vi "HealthCheck.vi"() -> ()   [LabVIEW 2017]
panel:
  out "Right Velocity":sgl
  out "BR Count":u8
  out "FR Count":u8
  in  "FPGA_Ref":T1
  in  "LOG":bool
  out "Reserve Battery Voltage 2":string
  out "IMU Z Accel":string
  out "IMU Y Accel":string
  out "IMU X Accel":string
  out "Light Sensor Right":string
  out "Light Sensor Left":string
  out "IR 4":string
  out "IR 3":string
  out "PCS Temp 2":string
  out "Pn High Pressure":string
  out "Pn Low Pressure":string
  out "Ambient Pressure":string
  out "Highest Battery Temp":string
  out "Reserve Battery Voltage":string
  out "Primary Battery 2 Voltage":string
  out "Primary Battery 1 Voltage":string
  in  "IMU_Ref":T2
  out "Y/N? 2":bool
  out "Ambient P Max 2":dbl
  out "Ambient P 2":dbl
  out "Downstream Right":dbl
  out "Y/N?":bool
  out "IMU Z Max":dbl
  out "IMU Z":dbl
  out "IMU Z Min":dbl
  out "Y/N? 3":bool
  out "IMU Y Max":dbl
  out "IMU Y":dbl
  out "IMU Y Min":dbl
  out "Y/N? 4":bool
  out "IMU X Max":dbl
  out "IMU X":dbl
  out "IMU X Min":dbl
  out "HP":dbl
  out "Y/N? 5":bool
  out "LS FR Max":dbl
  out "LS Right":dbl
  out "LS FR Min":dbl
  out "Y/N? 6":bool
  out "LS FL Max":dbl
  out "LS Left":dbl
  out "LS FL Min":dbl
  out "Y/N? 7":bool
  out "IR 2 Max":dbl
  out "IR 2":dbl
  out "IR 2 Min":dbl
  out "Y/N? 8":bool
  out "IR 1 Max":dbl
  out "IR 1":dbl
  out "IR 1 Min":dbl
  out "Y/N? 9":bool
  out "Ambient P Max":dbl
  out "Ambient P":dbl
  out "Ambient P Min":dbl
  out "Y/N? 10":bool
  out "LP Max":dbl
  out "LP":dbl
  out "LP1 Min":dbl
  out "Y/N? 11":bool
  out "HP Max":dbl
  out "HP Min":dbl
  out "Y/N? 12":bool
  out "PCS Temp Max":dbl
  out "PCS Temp":dbl
  out "PCS Temp Min":dbl
  out "Y/N? 13":bool
  out "HBT Max":dbl
  out "HBT":dbl
  out "HBT Min":dbl
  out "Y/N? 14":bool
  out "RBV Max":dbl
  out "RBV":dbl
  out "RBV Min":dbl
  out "Y/N? 15":bool
  out "PB2V Max":dbl
  out "PB2 V":dbl
  out "PB2V Min":dbl
  out "Y/N? 16":bool
  out "PB1V Max":dbl
  out "PB1V":dbl
  out "PB1V Min":dbl
  # "Sensor"
  # "Min"
  # "Actual"
  # "Max"
  # "Status"
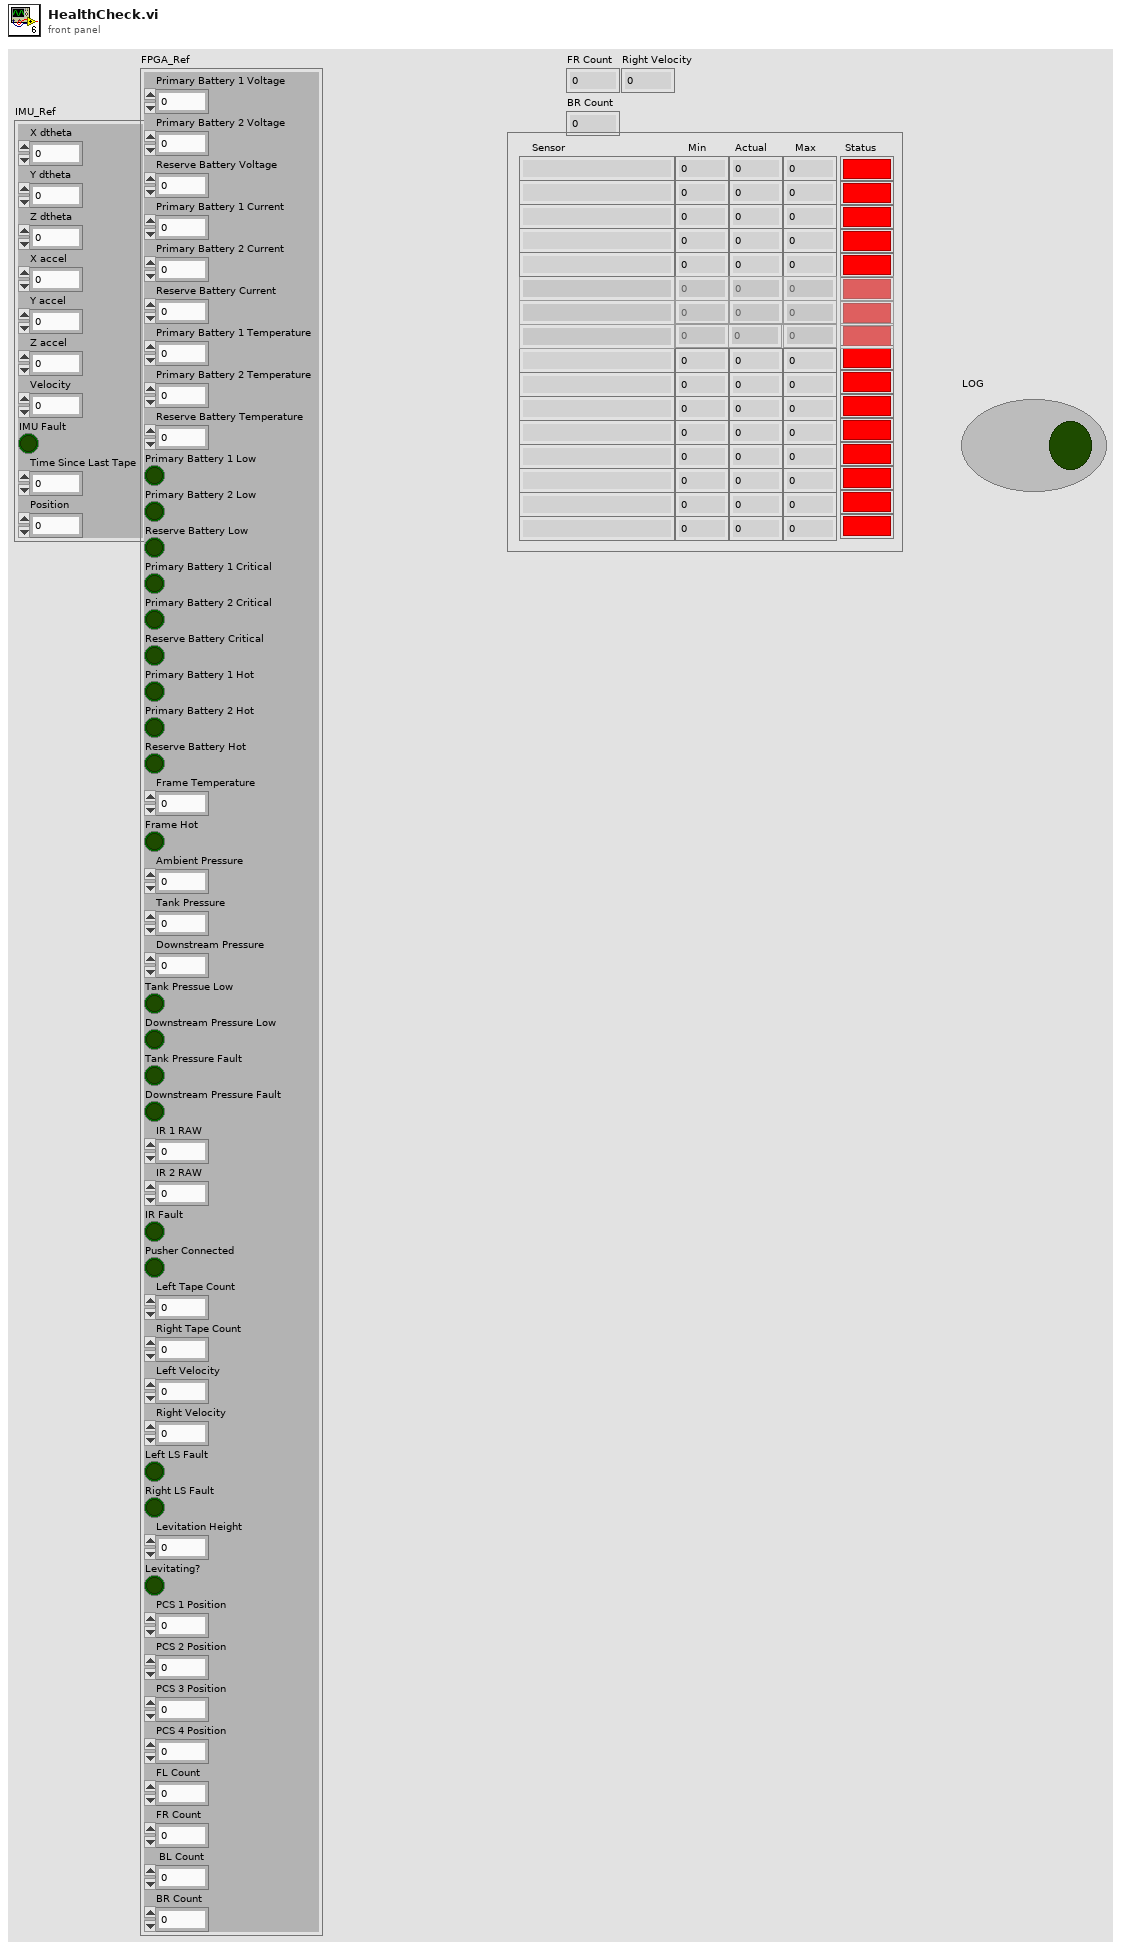
[diagram p1: front panel]
types:
  T1 = cluster{"Primary Battery 1 Voltage":sgl, "Primary Battery 2 Voltage":sgl, "Reserve Battery Voltage":sgl, "Primary Battery 1 Current":sgl, "Primary Battery 2 Current":sgl, "Reserve Battery Current":sgl, "Primary Battery 1 Temperature":sgl, "Primary Battery 2 Temperature":sgl, "Reserve Battery Temperature":sgl, "Primary Battery 1 Low":bool, "Primary Battery 2 Low":bool, "Reserve Battery Low":bool, "Primary Battery 1 Critical":bool, "Primary Battery 2 Critical":bool, "Reserve Battery Critical":bool, "Primary Battery 1 Hot":bool, "Primary Battery 2 Hot":bool, "Reserve Battery Hot":bool, "Frame Temperature":sgl, "Frame Hot":bool, "Ambient Pressure":sgl, "Tank Pressure":sgl, "Downstream Pressure":sgl, "Tank Pressue Low":bool, "Downstream Pressure Low":bool, "Tank Pressure Fault":bool, "Downstream Pressure Fault":bool, "IR 1 RAW":sgl, "IR 2 RAW":sgl, "IR Fault":bool, "Pusher Connected":bool, "Left Tape Count":u32, "Right Tape Count":u32, "Left Velocity":sgl, "Right Velocity":sgl, "Left LS Fault":bool, "Right LS Fault":bool, "Levitation Height":sgl, "Levitating?":bool, "PCS 1 Position":sgl, "PCS 2 Position":sgl, "PCS 3 Position":sgl, "PCS 4 Position":sgl, "FL Count":u8, "FR Count":u8, " BL Count":u8, "BR Count":u8}
  T2 = cluster{"X dtheta":sgl, "Y dtheta":sgl, "Z dtheta":sgl, "X accel":sgl, "Y accel":sgl, "Z accel":sgl, "Velocity":sgl, "IMU Fault":bool, "Time Since Last Tape":sgl, "Position":sgl}
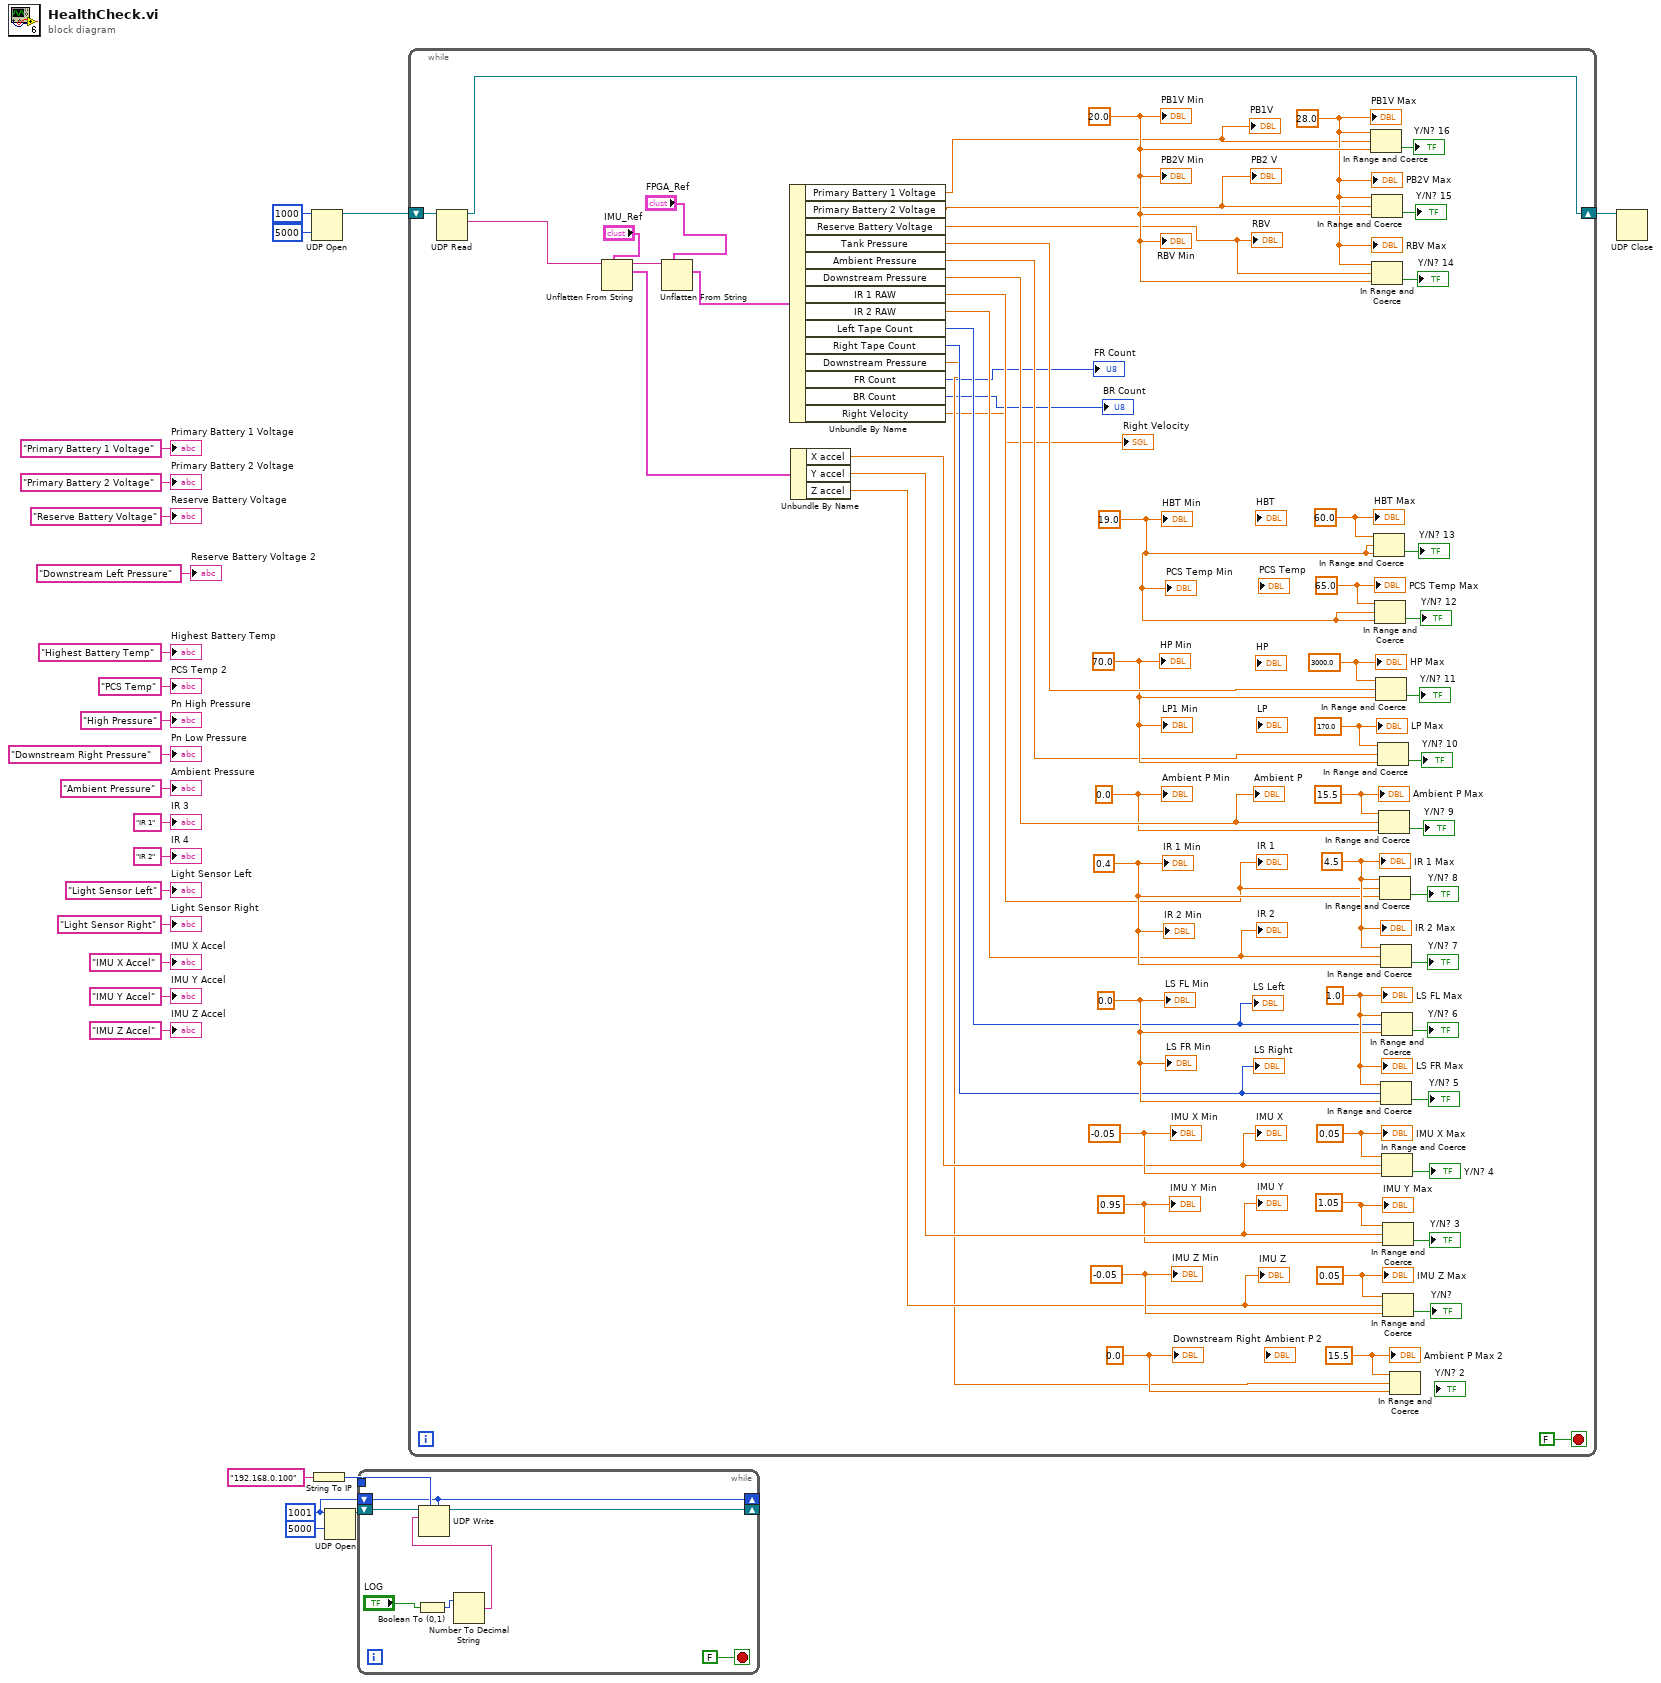
[diagram p0: block diagram]
diagram:
  w4 = u16 1001 ("port")
  n1 = UDP Open(9:5000 ("timeout ms (25000)"), 11:u16 1000 ("port")) -> (port=w25:refnum<k16>)  [unwired: 3 in, 2 out]
  n2 = String To IP(1:"192.168.0.100" ("name")) -> (0:w3:u32)
  n3 = UDP Open(9:5000 ("timeout ms (25000)"), 11:w4) -> (port=w5:refnum<k16>)  [unwired: 3 in, 2 out]
  n4 = while {
    tunnel: w3 -> [w32]
    shift-right: [w27] -> _
    shift-left: w5 -> [w33]
    shift-right: [w26] -> _
    shift-left: w4 -> [w26]
    stop <- FALSE stop-if-true
    n5 = Boolean To (0,1)(Boolean="LOG") -> (0, 1=w30:i16)
    n6 = Number To Decimal String(number=w30) -> (decimal integer string=w29:string)  [unwired: 1 in]
    n7 = UDP Write(address=w32, port or service name=w26, connection ID=w33, data in=w29) -> (3:w27:refnum<k16>)  [unwired: 2 in, 1 out]
  }
  n8 = while {
    shift-right: [w41] -> w6
    shift-left: w25 -> [w48]
    stop <- FALSE stop-if-true
    w38 = 1.05 ("IMU Z Max")
    w39 = 0.95 ("IMU X Min")
    w51 = 15.5 ("Ambient P Max")
    w50 = 0.0 ("Ambient P Min")
    w60 = 0.05 ("IMU Z Max")
    w62 = 0.05 ("IMU X Max")
    w58 = -0.05 ("IMU Z Min")
    w61 = -0.05 ("IMU X Min")
    w69 = 1.0 ("LS FL Max")
    w68 = 0.0 ("LS FL Min")
    w81 = 4.5 ("IR 1 Max")
    w80 = 0.4 ("IR 1 Min")
    w84 = 15.5 ("Ambient P Max")
    w82 = 0.0 ("Ambient P Min")
    w87 = 170.0 ("LP Max")
    w89 = 3000.0 ("HP Max")
    w86 = 70.0 ("HP Min")
    w90 = 65.0 ("PCS Temp")
    w91 = 60.0 ("HBT Max")
    w40 = 19.0 ("HBT Min")
    w93 = 28.0 ("PB1V Max")
    w94 = 20.0 ("PB1V Min")
    n9 = UDP Read(connection ID=w48) -> (data out=w47:string, 3:w41:refnum<k16>)  [unwired: 3 in, 3 out]
    n10 = Unflatten From String(type="IMU_Ref", binary string=w47) -> (rest of the binary string=w43:string, value=w45:T2)  [unwired: 3 in, 1 out]
    n11 = Unflatten From String(type="FPGA_Ref", binary string=w43) -> (value=w42:T1)  [unwired: 3 in, 2 out]
    n12 = Unbundle By Name(w42) -> ("Primary Battery 1 Voltage"=w54:sgl, "Primary Battery 2 Voltage"=w53:sgl, "Reserve Battery Voltage"=w52:sgl, "Tank Pressure"=w88:sgl, "Ambient Pressure"=w85:sgl, "Downstream Pressure"=w83:sgl, "IR 1 RAW"=w78:sgl, "IR 2 RAW"=w79:sgl, "Left Tape Count"=w65:u32, "Right Tape Count"=w67:u32, "Downstream Pressure"=w49:sgl, "FR Count"=→"FR Count":u8, "BR Count"=→"BR Count":u8, "Right Velocity"=→"Right Velocity":sgl)
    "PB1V" <- w54
    "PB2 V" <- w53
    "RBV" <- w52
    "Ambient P" <- w83
    "IR 1" <- w78
    "IR 2" <- w79
    "LS Left" <- w65
    "LS Right" <- w67
    n13 = Unbundle By Name(w45) -> ("X accel"=w57:sgl, "Y accel"=w55:sgl, "Z accel"=w56:sgl)
    "IMU X" <- w57
    "IMU Y" <- w55
    "IMU Z" <- w56
    n14 = In Range and Coerce(upper limit=w93, x=w54, lower limit=w94) -> (In Range?=→"Y/N? 16":bool)  [unwired: 1 out]
    n15 = In Range and Coerce(upper limit=w93, x=w53, lower limit=w94) -> (In Range?=→"Y/N? 15":bool)  [unwired: 1 out]
    n16 = In Range and Coerce(upper limit=w93, x=w52, lower limit=w94) -> (In Range?=→"Y/N? 14":bool)  [unwired: 1 out]
    n17 = In Range and Coerce(upper limit=w91, x=w40, lower limit=w40) -> (In Range?=→"Y/N? 13":bool)  [unwired: 1 out]
    n18 = In Range and Coerce(upper limit=w90, x=w40, lower limit=w40) -> (In Range?=→"Y/N? 12":bool)  [unwired: 1 out]
    n19 = In Range and Coerce(upper limit=w89, x=w88, lower limit=w86) -> (In Range?=→"Y/N? 11":bool)  [unwired: 1 out]
    n20 = In Range and Coerce(upper limit=w87, x=w85, lower limit=w86) -> (In Range?=→"Y/N? 10":bool)  [unwired: 1 out]
    n21 = In Range and Coerce(upper limit=w84, x=w83, lower limit=w82) -> (In Range?=→"Y/N? 9":bool)  [unwired: 1 out]
    n22 = In Range and Coerce(upper limit=w81, x=w78, lower limit=w80) -> (In Range?=→"Y/N? 8":bool)  [unwired: 1 out]
    n23 = In Range and Coerce(upper limit=w81, x=w79, lower limit=w80) -> (In Range?=→"Y/N? 7":bool)  [unwired: 1 out]
    n24 = In Range and Coerce(upper limit=w69, x=w67, lower limit=w68) -> (In Range?=→"Y/N? 5":bool)  [unwired: 1 out]
    n25 = In Range and Coerce(upper limit=w69, x=w65, lower limit=w68) -> (In Range?=→"Y/N? 6":bool)  [unwired: 1 out]
    n26 = In Range and Coerce(upper limit=w62, x=w57, lower limit=w61) -> (In Range?=→"Y/N? 4":bool)  [unwired: 1 out]
    n27 = In Range and Coerce(upper limit=w38, x=w55, lower limit=w39) -> (In Range?=→"Y/N? 3":bool)  [unwired: 1 out]
    n28 = In Range and Coerce(upper limit=w60, x=w56, lower limit=w58) -> (In Range?=→"Y/N?":bool)  [unwired: 1 out]
    n29 = In Range and Coerce(upper limit=w51, x=w49, lower limit=w50) -> ()  [unwired: 2 out]
    "PB1V Min" <- w94
    "PB1V Max" <- w93
    "PB2V Min" <- w94
    "PB2V Max" <- w93
    "RBV Min" <- w94
    "RBV Max" <- w93
    "HBT Min" <- w40
    "HBT Max" <- w91
    "PCS Temp Min" <- w40
    "PCS Temp Max" <- w90
    "HP Min" <- w86
    "HP Max" <- w89
    "LP1 Min" <- w86
    "LP Max" <- w87
    "Ambient P Min" <- w82
    "Ambient P Max" <- w84
    "IR 1 Min" <- w80
    "IR 1 Max" <- w81
    "IR 2 Min" <- w80
    "IR 2 Max" <- w81
    "LS FL Min" <- w68
    "LS FL Max" <- w69
    "LS FR Min" <- w68
    "LS FR Max" <- w69
    "IMU X Min" <- w61
    "IMU X Max" <- w62
    "IMU Y Min" <- w39
    "IMU Y Max" <- w38
    "IMU Z Min" <- w58
    "IMU Z Max" <- w60
    "Downstream Right" <- w50
    "Ambient P Max 2" <- w51
  }
  n30 = UDP Close(connection ID=w6) -> ()  [unwired: 1 in, 2 out]
  "Primary Battery 1 Voltage" <- "Primary Battery 1 Voltage" ("Primary Battery 1 Voltage")
  "Primary Battery 2 Voltage" <- "Primary Battery 2 Voltage" ("Primary Battery 2 Voltage")
  "Reserve Battery Voltage" <- "Reserve Battery Voltage" ("Reserve Battery Voltage")
  "Highest Battery Temp" <- "Highest Battery Temp" ("Highest Battery Temp")
  "Ambient Pressure" <- "Ambient Pressure" ("Ambient Pressure")
  "Pn Low Pressure" <- "Downstream Right Pressure" ("Pn Low Pressure")
  "Pn High Pressure" <- "High Pressure" ("Pn High Pressure")
  "PCS Temp 2" <- "PCS Temp" ("PCS Temp")
  "IR 3" <- "IR 1" ("IR 1")
  "IR 4" <- "IR 2" ("IR 2")
  "Light Sensor Left" <- "Light Sensor Left" ("Light Sensor FL")
  "Light Sensor Right" <- "Light Sensor Right" ("Light Sensor FR")
  "IMU X Accel" <- "IMU X Accel" ("IMU X Accel")
  "IMU Y Accel" <- "IMU Y Accel" ("IMU Y Accel")
  "IMU Z Accel" <- "IMU Z Accel" ("IMU Z Accel")
  "Reserve Battery Voltage 2" <- "Downstream Left Pressure" ("Reserve Battery Voltage")
